vi "ConnectandDisconnect.vi"(0 "Virtual Device Name":string="SwitchConfiguration1", 1 "Connection Specification (\"\")":string, 2 "Disconnection Specification (\"\")":string, 5 "Option String (\"\")":string, 11 "error in":errorcluster {"code" format="%.0x"}) -> (15 "error out":errorcluster {"code" format="%.0x"})   [LabVIEW 2021]
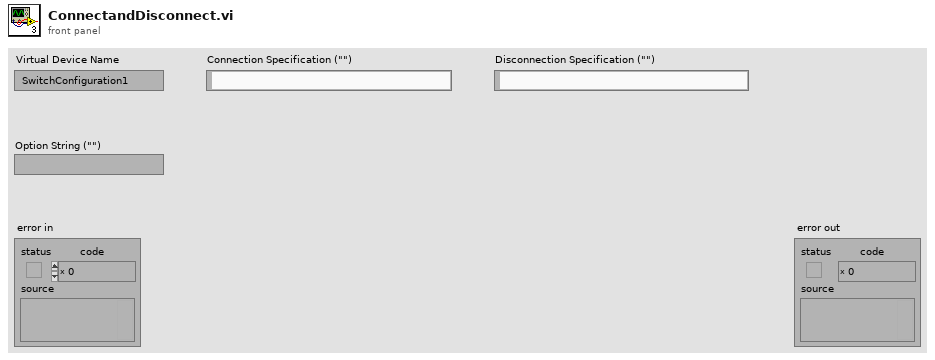
[diagram p1: front panel]
types:
  T1 = typedef "niSE SessionRefnum.ctl" = refnum<k1>
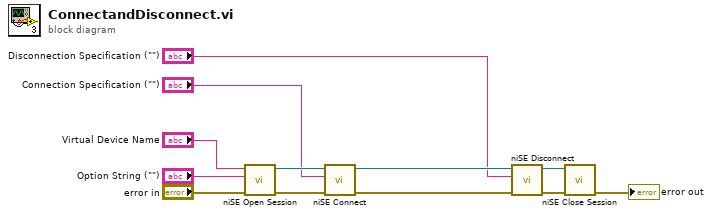
[diagram p0: block diagram]
diagram:
  n1 = call <vilib>:"niSE Open Session.vi"("error in (no error)"="error in", "Option String (\"\")"="Option String (\"\")", "Virtual Device Name (SwitchConfiguration1)"="Virtual Device Name") -> ("error out"=w9:errorcluster, "NISE Session (out)"=w12:T1)  [unwired: 3 in]
  n2 = call <vilib>:"niSE Connect.vi"("error in (no error)"=w9, "Connection Specification (\"\")"="Connection Specification (\"\")", "NISE Session (in)"=w12) -> ("error out"=w8:errorcluster, "NISE Session (out)"=w11:T1)  [unwired: 7 in]
  n3 = call <vilib>:"niSE Disconnect.vi"("error in (no error)"=w8, "Disconnection Specification (\"\")"="Disconnection Specification (\"\")", "NISE Session (in)"=w11) -> ("error out"=w7:errorcluster, "NISE Session (out)"=w10:T1)  [unwired: 3 in]
  n4 = call <vilib>:"niSE Close Session.vi"("error in (no error)"=w7, "NISE Session (in)"=w10) -> ("error out"=→"error out":errorcluster)  [unwired: 5 in]
